vi "Structure to Supercell Structure.vi"(8 "c lattice factor":i16=1 min=1 max=1000, 9 "b lattice factor":i16=1 min=1 max=1000, 10 "a lattice factor":i16=1 min=1 max=1000, 11 "Input Structure":T1={"Structure Name"="A3B3_twin", "Lattice vector a"=[4.67354, 0.0, 0.0], "Lattice vector b"=[0.0, 8.0948, 0.0], "Lattice vector c"=[0.0, 0.0, 22.8956], "Atoms Array"=[{"Atom Name"="Cd", "Positions (Direct)"=[[0.0, 0.3333160110632741, 0.0416917449166463], [0.5000009999999975, 0.8333170110632716, 0.0416917449166463], [0.5000009999999975, 0.1666621408709168, 0.208337818520255], [0.0, 0.6666631408709214, 0.208337818520255], [0.0, 8.4662249422e-06, 0.3749383421346864], [0.5000009999999975, 0.5000094662249397, 0.3749383421346864], [0.0, -8.4662249422e-06, 0.8749383421346864], [0.5000009999999975, 0.4999925337750553, 0.8749383421346864], [0.0, 0.3333388591290807, 0.7083368185202576], [0.5000009999999975, 0.8333398591290782, 0.7083368185202576], [0.5000009999999975, 0.1666849889367233, 0.5416917449166463], [0.0, 0.6666859889367279, 0.5416917449166463]], "Positions (Cartesian)"=[[0.0, 2.6981264463549905, 0.9545575149135672], [2.3367746735399884, 6.745534541154971, 0.9545575149135672], [2.3367746735399884, 1.3490966979218972, 4.770019357712351], [0.0, 5.396504792721934, 4.770019357712351], [0.0, 6.853239766212056e-05, 8.584438306178926], [2.3367746735399884, 4.047476627197642, 8.584438306178926], [0.0, -6.853239766212056e-05, 20.032238306178925], [2.3367746735399884, 4.047339562402318, 20.032238306178925], [0.0, 2.698311396878082, 16.217796462112414], [2.3367746735399884, 6.745719491678061, 16.217796462112414], [2.3367746735399884, 1.3492816484449877, 12.402357514913568], [0.0, 5.396689743245025, 12.402357514913568]]}, {"Atom Name"="Te", "Positions (Direct)"=[[0.0, -2.2822775934e-06, 0.0001327438415307], [0.5000009999999975, 0.499998717722404, 0.0001327438415307], [0.0, 0.3333991470731503, 0.166602258546053], [0.5000009999999975, 0.8334001470731478, 0.166602258546053], [0.5000009999999975, 0.1666248769120535, 0.3332990920408234], [0.0, 0.6666258769120581, 0.3332990920408234], [0.0, 0.333376123087944, 0.8332980920408259], [0.5000009999999975, 0.8333771230879414, 0.8332980920408259], [0.5000009999999975, 0.1666018529268472, 0.6666022585460529], [0.0, 0.6666028529268517, 0.6666022585460529], [0.0, 2.2822775934e-06, 0.5001327438415307], [0.5000009999999975, 0.5000032822775909, 0.5001327438415307]], "Positions (Cartesian)"=[[0.0, -1.8474580663054318e-05, 0.003039249898150295], [2.3367746735399884, 4.047389620219316, 0.003039249898150295], [0.0, 2.698799415727737, 3.814458670767012], [2.3367746735399884, 6.746207510527716, 3.814458670767012], [2.3367746735399884, 1.3487950536276905, 7.631082691729877], [0.0, 5.396203148427728, 7.631082691729877], [0.0, 2.698613041172289, 19.078859796129937], [2.3367746735399884, 6.746021135972268, 19.078859796129937], [2.3367746735399884, 1.3486086790722427, 15.262258670767011], [0.0, 5.396016773872279, 15.262258670767011], [0.0, 1.8474580663054318e-05, 11.450839249898152], [2.3367746735399884, 4.047426569380643, 11.450839249898152]]}], "# of atoms"=24}) -> (3 "Supercell Structure":T1={"Structure Name"="A3B3_twin", "Lattice vector a"=[4.67354, 0.0, 0.0], "Lattice vector b"=[0.0, 8.0948, 0.0], "Lattice vector c"=[0.0, 0.0, 22.8956], "Atoms Array"=[{"Atom Name"="Cd", "Positions (Direct)"=[[0.0, 0.3333160110632741, 0.0416917449166463], [0.5000009999999975, 0.8333170110632716, 0.0416917449166463], [0.5000009999999975, 0.1666621408709168, 0.208337818520255], [0.0, 0.6666631408709214, 0.208337818520255], [0.0, 8.4662249422e-06, 0.3749383421346864], [0.5000009999999975, 0.5000094662249397, 0.3749383421346864], [0.0, -8.4662249422e-06, 0.8749383421346864], [0.5000009999999975, 0.4999925337750553, 0.8749383421346864], [0.0, 0.3333388591290807, 0.7083368185202576], [0.5000009999999975, 0.8333398591290782, 0.7083368185202576], [0.5000009999999975, 0.1666849889367233, 0.5416917449166463], [0.0, 0.6666859889367279, 0.5416917449166463]], "Positions (Cartesian)"=[[0.0, 2.6981264463549905, 0.9545575149135672], [2.3367746735399884, 6.745534541154971, 0.9545575149135672], [2.3367746735399884, 1.3490966979218972, 4.770019357712351], [0.0, 5.396504792721934, 4.770019357712351], [0.0, 6.853239766212056e-05, 8.584438306178926], [2.3367746735399884, 4.047476627197642, 8.584438306178926], [0.0, -6.853239766212056e-05, 20.032238306178925], [2.3367746735399884, 4.047339562402318, 20.032238306178925], [0.0, 2.698311396878082, 16.217796462112414], [2.3367746735399884, 6.745719491678061, 16.217796462112414], [2.3367746735399884, 1.3492816484449877, 12.402357514913568], [0.0, 5.396689743245025, 12.402357514913568]]}, {"Atom Name"="Te", "Positions (Direct)"=[[0.0, -2.2822775934e-06, 0.0001327438415307], [0.5000009999999975, 0.499998717722404, 0.0001327438415307], [0.0, 0.3333991470731503, 0.166602258546053], [0.5000009999999975, 0.8334001470731478, 0.166602258546053], [0.5000009999999975, 0.1666248769120535, 0.3332990920408234], [0.0, 0.6666258769120581, 0.3332990920408234], [0.0, 0.333376123087944, 0.8332980920408259], [0.5000009999999975, 0.8333771230879414, 0.8332980920408259], [0.5000009999999975, 0.1666018529268472, 0.6666022585460529], [0.0, 0.6666028529268517, 0.6666022585460529], [0.0, 2.2822775934e-06, 0.5001327438415307], [0.5000009999999975, 0.5000032822775909, 0.5001327438415307]], "Positions (Cartesian)"=[[0.0, -1.8474580663054318e-05, 0.003039249898150295], [2.3367746735399884, 4.047389620219316, 0.003039249898150295], [0.0, 2.698799415727737, 3.814458670767012], [2.3367746735399884, 6.746207510527716, 3.814458670767012], [2.3367746735399884, 1.3487950536276905, 7.631082691729877], [0.0, 5.396203148427728, 7.631082691729877], [0.0, 2.698613041172289, 19.078859796129937], [2.3367746735399884, 6.746021135972268, 19.078859796129937], [2.3367746735399884, 1.3486086790722427, 15.262258670767011], [0.0, 5.396016773872279, 15.262258670767011], [0.0, 1.8474580663054318e-05, 11.450839249898152], [2.3367746735399884, 4.047426569380643, 11.450839249898152]]}], "# of atoms"=24})   [LabVIEW 2010]
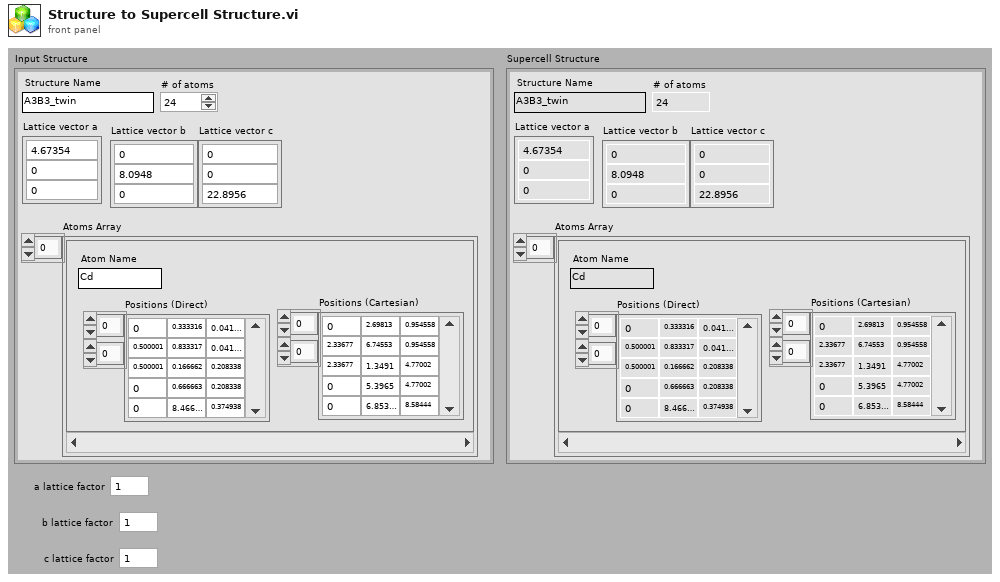
[diagram p1: front panel]
types:
  T1 = cluster{"Structure Name":string, "Lattice vector a":dbl[], "Lattice vector b":dbl[], "Lattice vector c":dbl[], "Atoms Array":cluster{"Atom Name":string, "Positions (Direct)":dbl[][], "Positions (Cartesian)":dbl[][]}[], "# of atoms":i32}
  T2 = cluster{"Atom Name":string, "Positions (Direct)":dbl[][], "Positions (Cartesian)":dbl[][]}[]
  T3 = cluster{"Atom Name":string, "Positions (Direct)":dbl[][], "Positions (Cartesian)":dbl[][]}
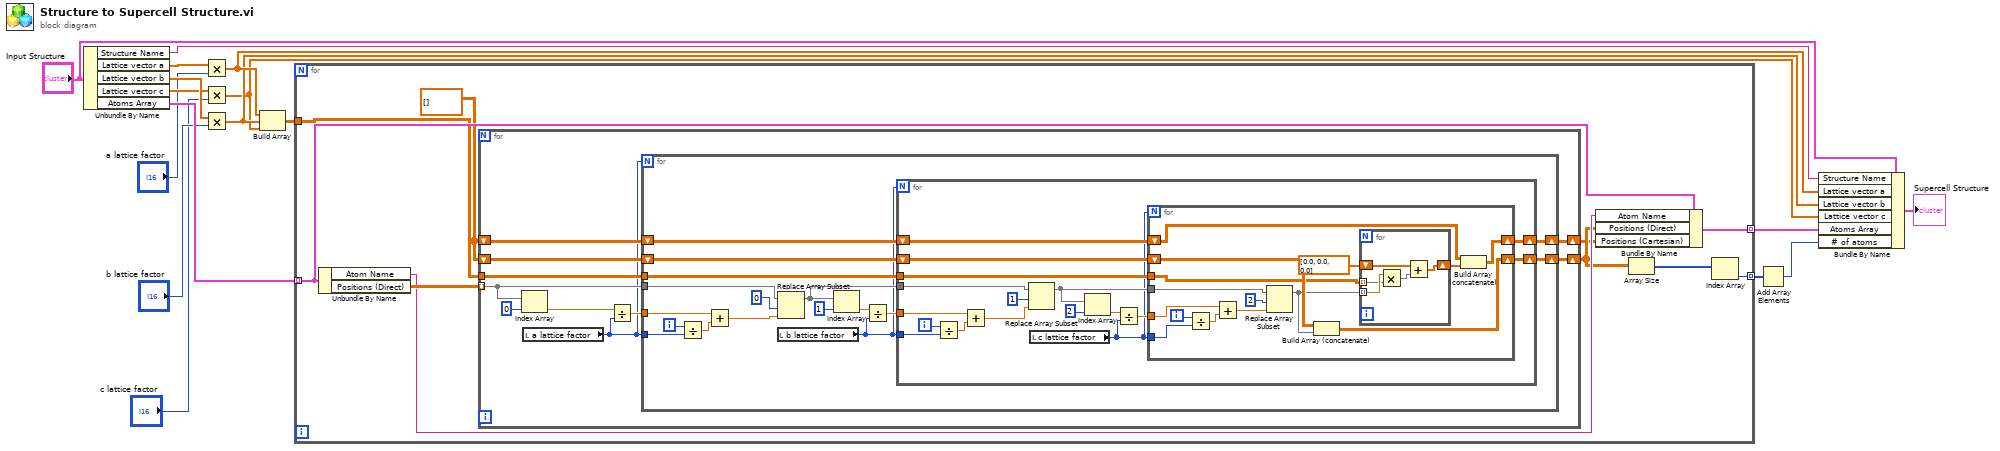
[diagram p0: block diagram]
diagram:
  n1 = Unbundle By Name("Input Structure") -> ("Structure Name"=w13:string, "Lattice vector a"=w16:dbl[], "Lattice vector b"=w12:dbl[], "Lattice vector c"=w11:dbl[], "Atoms Array"=w17:T2)
  n2 = Multiply(x=w16, y="a lattice factor") -> (x*y=w4:dbl[])
  n3 = Multiply(x=w11, y="c lattice factor") -> (x*y=w2:dbl[])
  n4 = Multiply(x=w12, y="b lattice factor") -> (x*y=w3:dbl[])
  n5 = Build Array(w4, w3, w2) -> (w1:dbl[][])
  n6 = for {
    tunnel: w17 -> [w26] mode=indexing
    tunnel: [w25] -> w7 mode=indexing
    tunnel: [w21] -> w6 mode=indexing
    tunnel: w1 -> [w20]
    w19 = dbl[][] []
    n7 = Unbundle By Name(w26) -> ("Atom Name"=w24:string, "Positions (Direct)"=w27:dbl[][])
    n8 = for {
      tunnel: w27 -> [w35] mode=indexing
      shift-right: [w33] -> w23
      shift-left: w19 -> [w32]
      tunnel: w20 -> [w31]
      shift-right: [w30] -> w18
      shift-left: w19 -> [w29]
      n9 = Index Array(array=w35, index=0) -> (element=w37:dbl)
      n10 = local read "a lattice factor"() -> (w28:i16)
      n11 = Divide(x=w37, y=w28) -> (x/y=w36:dbl)
      n12 = for {
        N: w28 -> [_]
        tunnel: w36 -> [w43]
        tunnel: w35 -> [w54]
        shift-right: [w48] -> w33
        shift-left: w32 -> [w47]
        tunnel: w31 -> [w46]
        shift-right: [w45] -> w30
        shift-left: w29 -> [w44]
        tunnel: w28 -> [w42]
        i -> [w39]
        n13 = Divide(x=w39, y=w42) -> (x/y=w41:dbl)
        n14 = Add(x=w43, y=w41) -> (x+y=w40:dbl)
        n15 = local read "b lattice factor"() -> (w38:i16)
        n16 = Replace Array Subset(array=w54, new element=w40, index=0) -> (w49:dbl[])
        n17 = Index Array(array=w49, index=1) -> (element=w50:dbl)
        n18 = Divide(x=w50, y=w38) -> (x/y=w52:dbl)
        n19 = for {
          N: w38 -> [_]
          tunnel: w52 -> [w57]
          tunnel: w49 -> [w67]
          shift-right: [w65] -> w48
          shift-left: w47 -> [w64]
          tunnel: w46 -> [w63]
          shift-right: [w62] -> w45
          shift-left: w44 -> [w61]
          tunnel: w38 -> [w58]
          i -> [w59]
          n20 = Divide(x=w59, y=w58) -> (x/y=w60:dbl)
          n21 = Add(x=w57, y=w60) -> (x+y=w56:dbl)
          n22 = Replace Array Subset(array=w67, new element=w56, index=1) -> (w66:dbl[])
          n23 = local read "c lattice factor"() -> (w55:i16)
          n24 = Index Array(array=w66, index=2) -> (element=w68:dbl)
          n25 = Divide(x=w68, y=w55) -> (x/y=w70:dbl)
          n26 = for {
            N: w55 -> [_]
            tunnel: w70 -> [w73]
            tunnel: w66 -> [w86]
            shift-right: [w84] -> w65
            shift-left: w64 -> [w83]
            tunnel: w63 -> [w81]
            shift-right: [w78] -> w62
            shift-left: w61 -> [w77]
            tunnel: w55 -> [w74]
            i -> [w75]
            n27 = Divide(x=w75, y=w74) -> (x/y=w76:dbl)
            n28 = Add(x=w73, y=w76) -> (x+y=w72:dbl)
            n29 = Replace Array Subset(array=w86, new element=w72, index=2) -> (w82:dbl[])
            n30 = Build Array (concatenate)(w83, w82) -> (w84:dbl[][])
            n31 = for {
              tunnel: w82 -> [w91] mode=indexing
              tunnel: w81 -> [w90] mode=indexing
              shift-right: [w88] -> w79
              shift-left: dbl[] [0.0, 0.0, 0.0] -> [w87]
              n32 = Multiply(x=w91, y=w90) -> (x*y=w89:dbl[])
              n33 = Add(x=w87, y=w89) -> (x+y=w88:dbl[])
            }
            n34 = Build Array (concatenate)(w77, w79) -> (w78:dbl[][])
          }
        }
      }
    }
    n35 = Bundle By Name(cluster=w26, "Atom Name"=w24, "Positions (Direct)"=w23, "Positions (Cartesian)"=w18) -> (w25:T3)
    n36 = Array Size(array=w23) -> (size(s)=w22:i32[])
    n37 = Index Array(array=w22) -> (element=w21:i32)  [unwired: 1 in]
  }
  n38 = Add Array Elements(numeric array=w6) -> (sum=w5:i32)
  n39 = Bundle By Name(cluster="Input Structure", "Structure Name"=w13, "Lattice vector a"=w4, "Lattice vector b"=w3, "Lattice vector c"=w2, "Atoms Array"=w7, "# of atoms"=w5) -> (→"Supercell Structure":T1)
